vi "theOne_V3.vi"() -> ()   [LabVIEW 2021]
uses:
  <userlib>/er4commlib_labview/er4commlib_labview.lvlib
  <resource>/objmgr/nicontrollersysapi.rc
  <vilib>/nisyscfg/nisyscfg.lvlib
  <resource>/objmgr/nisysapi.rc
panel:
  in  "Tab Control 2":enum32{"const", "tri", "squa", "steps"}(tab)
  in  "Voltage Stimulus const":cluster{"stimulus":bool, "Vhold [mV]":dbl}={"stimulus"=FALSE, "Vhold [mV]"=-50.0} {"Vhold [mV]" format="%_5f"}
  in  "Voltage Stimulus tri":T1={"stimulus"=FALSE, "Vhold [mV]"=-50.0, "Vamp [mV]"=0.0, "Thold [ms]"=0.0} {"Thold [ms]" format="%_5f"; "Vamp [mV]" format="%_5f"; "Vhold [mV]" format="%_5f"}
  in  "Voltage Stimulus squa":T2={"stimulus"=FALSE, "Vhold [mV]"=-50.0, "Vpulse [mV]"=0.0, "Thold [ms]"=0.0, "Tpulse [ms]"=200.0} {"Tpulse [ms]" format="%_5f"; "Thold [ms]" format="%_5f"; "Vpulse [mV]" format="%_5f"; "Vhold [mV]" format="%_5f"}
  in  "Voltage Stimulus steps":T3={"stimulus"=FALSE, "Vhold [mV]"=-50.0, "Vpulse [mV]"=0.0, "Vstep [mV]"=10.0, "N"=10, "Thold [ms]"=0.0, "Tpulse [ms]"=200.0, "testVoff [mV]"=200.0, "testVoffCh"=127} {"testVoff [mV]" format="%_5f"; "Tpulse [ms]" format="%_5f"; "Thold [ms]" format="%_5f"; "Vstep [mV]" format="%_5f"; "Vpulse [mV]" format="%_5f"; "Vhold [mV]" format="%_5f"}
  out "Array 6":dbl[][](array[numeric])
  in  "save!":bool=TRUE
  out "actuall saving path":path
  out "refTxtSave":refnum<file>
  out "saving?":bool
  out "System Resources:Memory:Free Virtual":dbl=30432984.0
  in  "Target (localhost)":refnum<k21>="localhost"
  out "# elements to save":i32=45
  out "# elements to display":i32
  in  "save to":path=path "C:/temp/test.txt"
  out "DataCh1":dbl[](graph)
  out "DataCh2":dbl[](graph)
  out "DataCh3":dbl[](graph)
  out "DataCh4":dbl[](graph)
  out "VolAndTrig":dbl[][](graph)
  out "triggerImage":picture
  in  "path to triggerImage file jpg":path=path "C:/neoDiag/MrAnderson/Img/trigger.jpg"
  in  "Trigger":T4={"manual start"=FALSE, "duration [us]"=200.0, "period [ms]"=1.0, "delay [us]"=0.0, "reps"=1000, "active"=TRUE} {"delay [us]" format="%_5f"; "period [ms]" format="%_5f"; "duration [us]" format="%_5f"}
  in  "acquire data":bool
  in  "stop":bool
  out "pulseTrainImage":picture
  in  "path to pulseTrainImage file jpg":path=path "C:/neoDiag/MrAnderson/Img/volProtVarAmpl.jpg"
  in  "Tab Control":enum32{"AcqPara", "AdvPara"}(tab)
  in  "Acquisition Parameters":T5={"Camera "=FALSE, "Period [ms]"=200.0, "Duration [ms]"=0.2, "Delay [ms]"=0.0, "Pulses [#]"=10, "sampling rate [kHz]"="1,25", "current range [nA]"="2", "time display [s]"=0.5, "time recording [s]"=0.0} {"Delay [ms]" format="%_5f"; "Duration [ms]" format="%_5f"; "Period [ms]" format="%_5f"}
  in  "advancedSettings":T6={"Channels to read"=6, " dataPackets to read"=100, "displayRange"=625, "time acq loop [ms]"=25, "time rest loop [ms]"=25}
  out "Error Out Int":u32
  out "Error Out String":string="clean"
  out "E4 parameters":T7={"currentChannelsNum out"=1, "voltageChannelsNum out"=4, "gpChannelsNum out"=1, "sampling rate [kHz]"=1.25, "real sampling rate [kHz]"=1.220703125, "Ch_min"=-2.0, "Ch_max"=2.0, "Ch_step"=6.103701895199438e-05, "Ch_unit"=1e-09}
  in  "Display 1":cluster{"ChArray":bool[]}={"ChArray"=[FALSE, TRUE, TRUE, TRUE, FALSE, FALSE]}
  out "Error Read":errorcluster
  # "8MBit per element\ncan be improved setting min buffer of readData.vi"
  # "DataCh1"
  # "DataCh2"
  # "DataCh3"
  # "DataCh4"
  # "Voltage"
  # "Trigger"
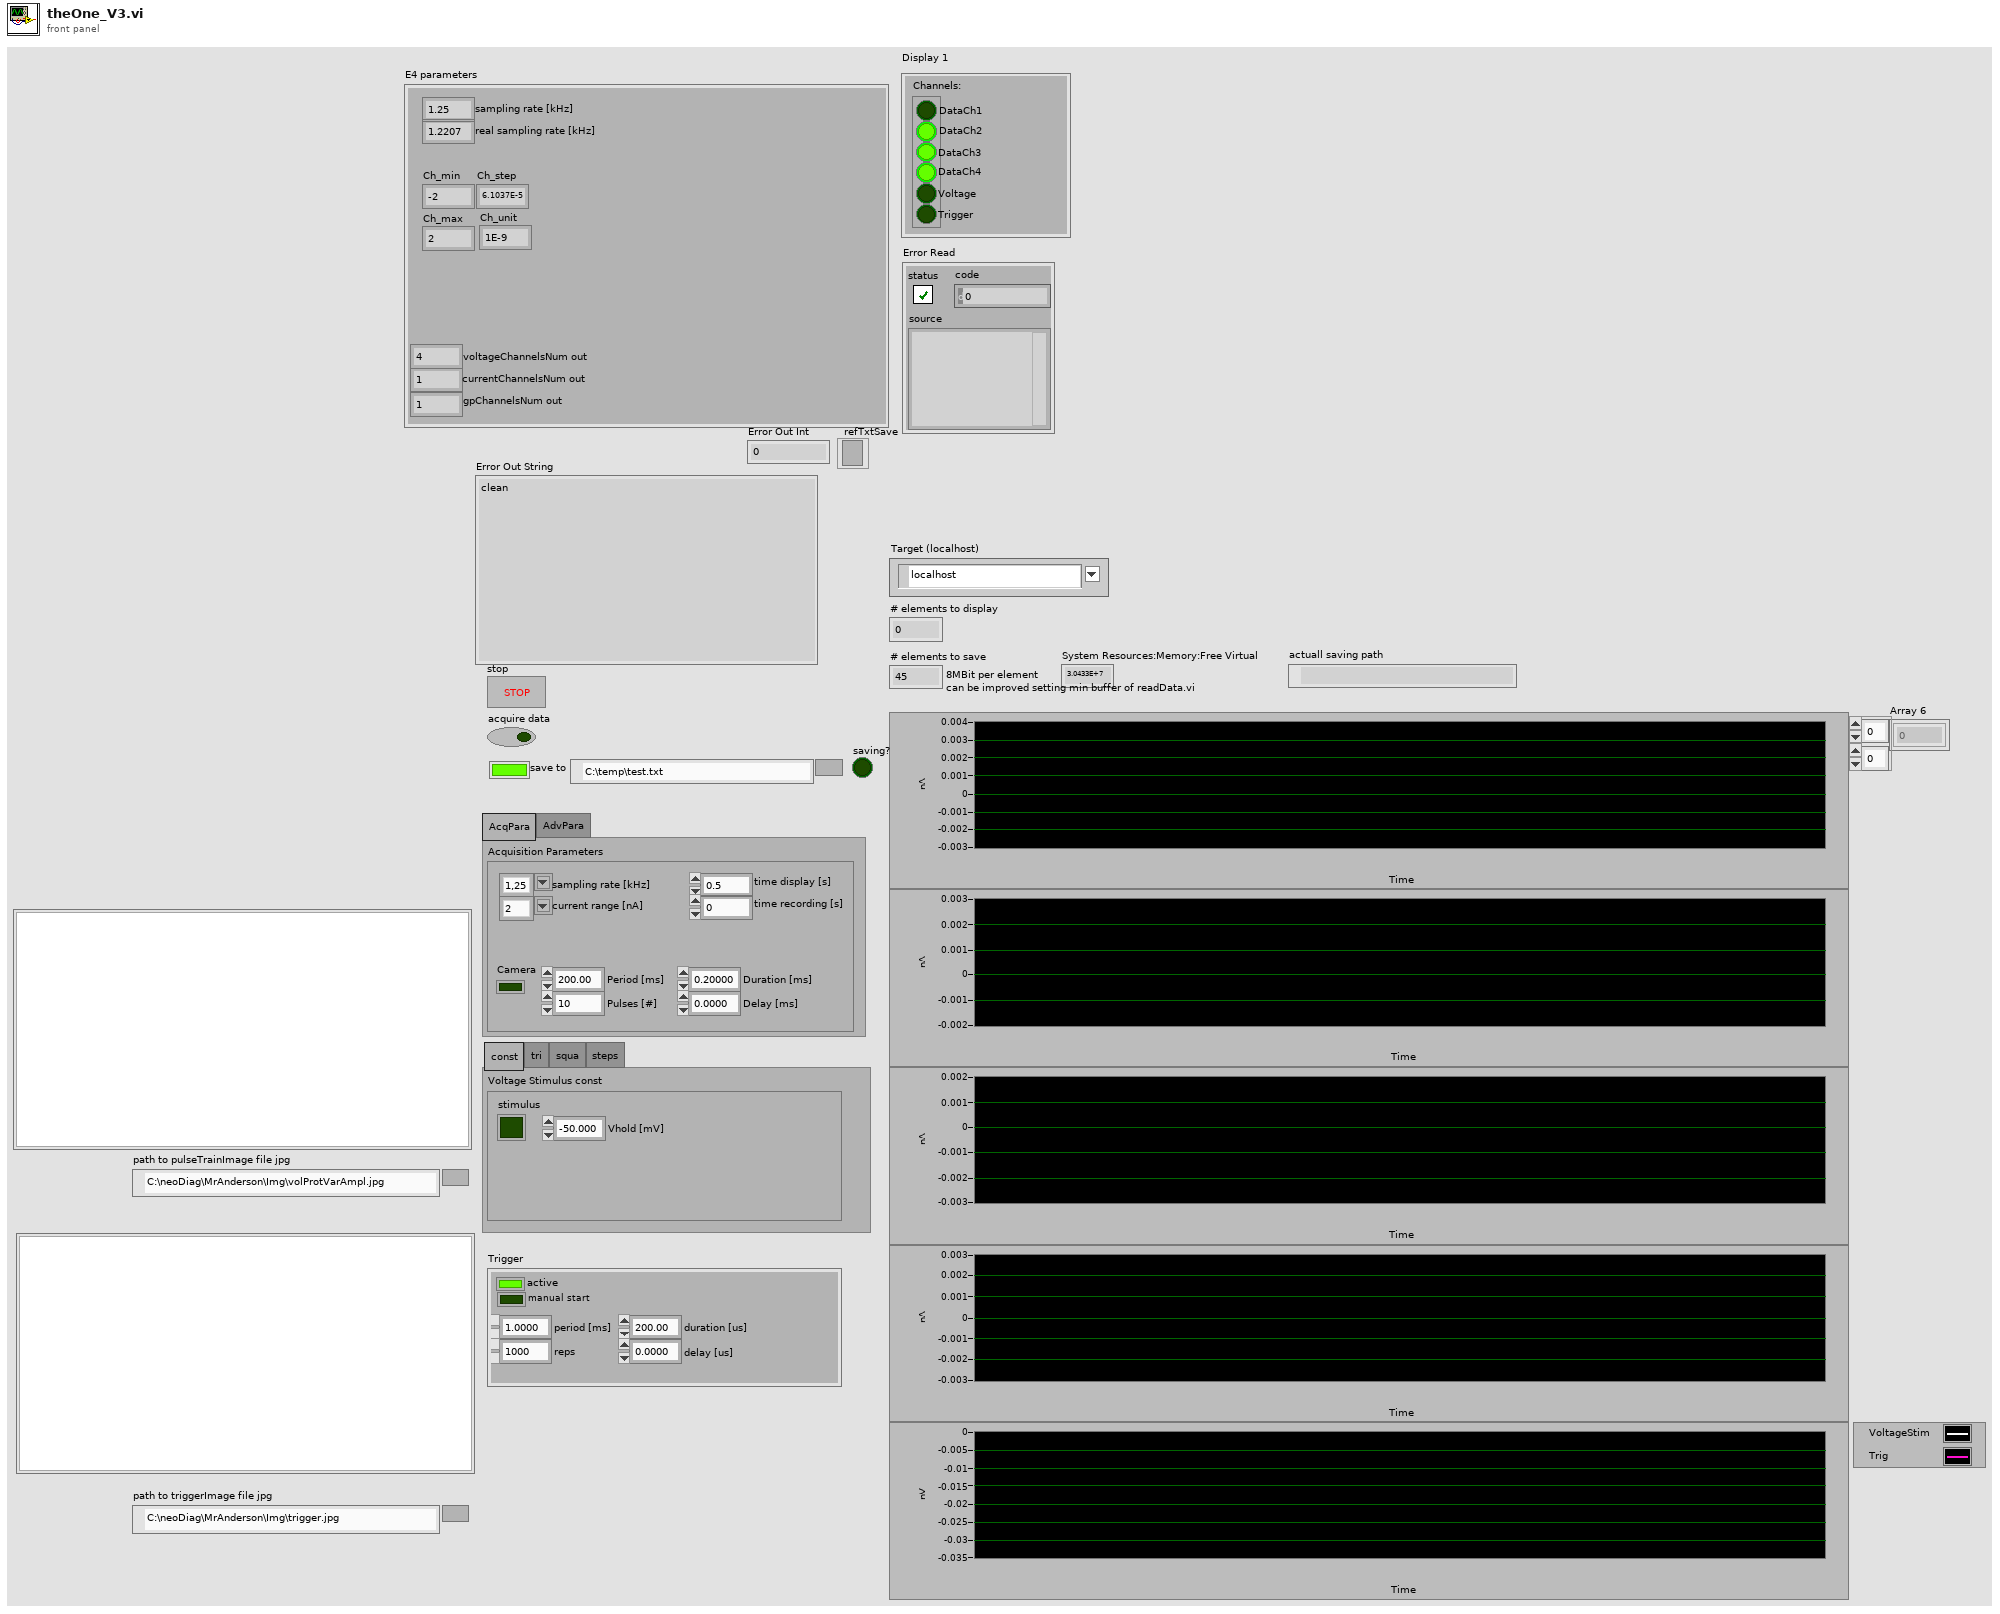
[diagram p1: front panel]
types:
  T1 = cluster{"stimulus":bool, "Vhold [mV]":dbl, "Vamp [mV]":dbl, "Thold [ms]":dbl}
  T2 = cluster{"stimulus":bool, "Vhold [mV]":dbl, "Vpulse [mV]":dbl, "Thold [ms]":dbl, "Tpulse [ms]":dbl}
  T3 = cluster{"stimulus":bool, "Vhold [mV]":dbl, "Vpulse [mV]":dbl, "Vstep [mV]":dbl, "N":u32, "Thold [ms]":dbl, "Tpulse [ms]":dbl, "testVoff [mV]":dbl, "testVoffCh":i8}
  T4 = cluster{"manual start":bool, "duration [us]":dbl, "period [ms]":dbl, "delay [us]":dbl, "reps":u32, "active":bool}
  T5 = cluster{"Camera ":bool, "Period [ms]":dbl, "Duration [ms]":dbl, "Delay [ms]":dbl, "Pulses [#]":u32, "sampling rate [kHz]":string, "current range [nA]":string, "time display [s]":dbl, "time recording [s]":dbl}
  T6 = cluster{"Channels to read":i32, " dataPackets to read":i32, "displayRange":i32, "time acq loop [ms]":u32, "time rest loop [ms]":u32}
  T7 = cluster{"currentChannelsNum out":u32, "voltageChannelsNum out":u32, "gpChannelsNum out":u32, "sampling rate [kHz]":dbl, "real sampling rate [kHz]":dbl, "Ch_min":dbl, "Ch_max":dbl, "Ch_step":dbl, "Ch_unit":dbl}
  T8 = cluster{"availableDataPackets":u32, "bufferOverflowFlag":bool, "lostDataFlag":bool, "saturationFlag":bool, "currentRangeIncreaseFlag":bool, "currentRangeDecreaseFlag":bool, "communicationErrorFlag":bool}
  T9 = enum16{"open", "replace", "create", "open or create", "replace or create", "replace or create with confirmation"}
  T10 = typedef "imagedata.ctl" = cluster{"image type":i32, "image depth":i32, "image":u8[], "mask":u8[], "colors":u32[], "Rectangle":cluster{"left":i16, "top":i16, "right":i16, "bottom":i16}}
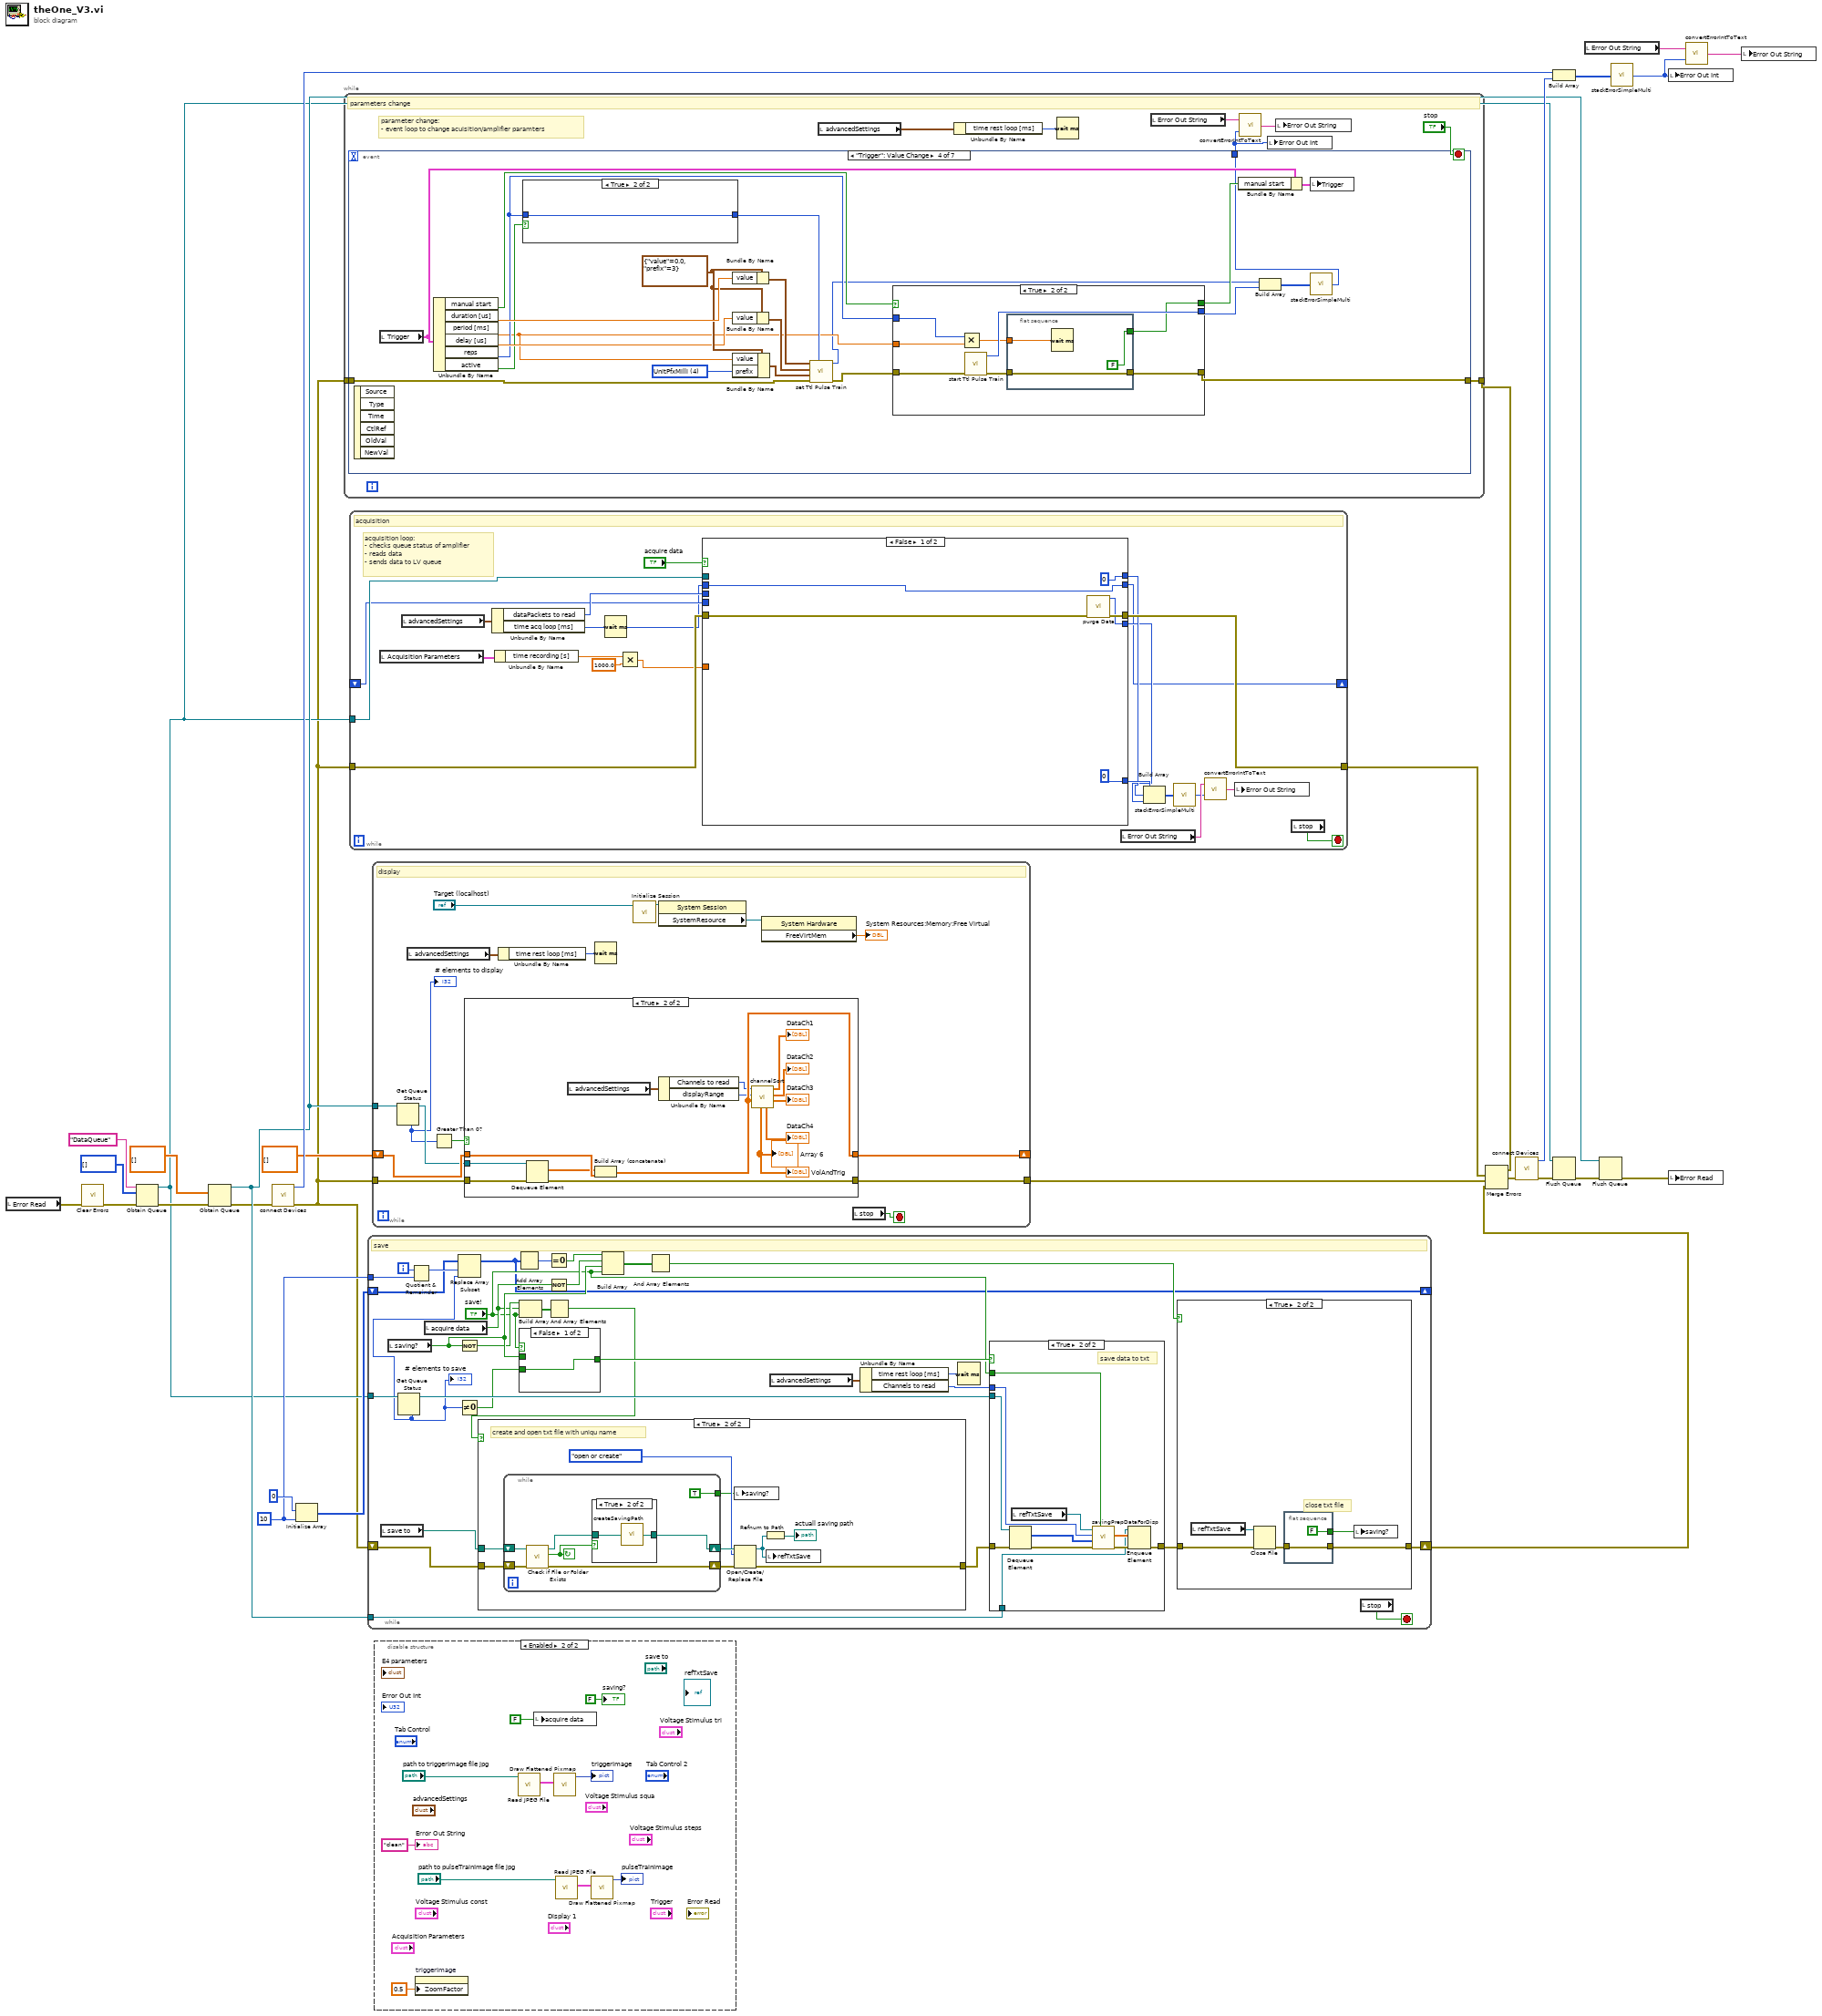
[diagram p0: block diagram]
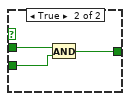
[diagram p2: hidden frame]
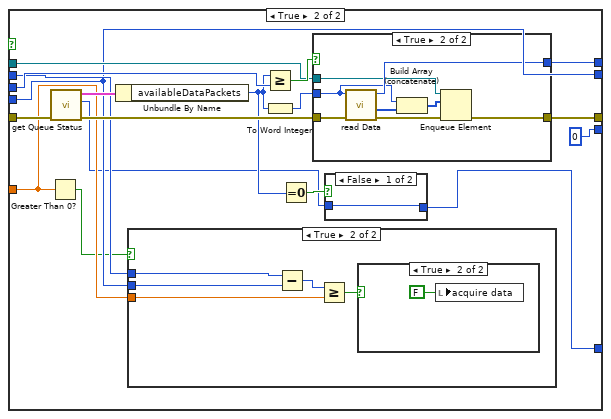
[diagram p8: hidden frame]
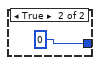
[diagram p9: hidden frame]
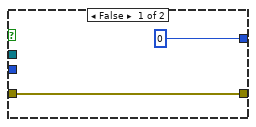
[diagram p12: hidden frame]
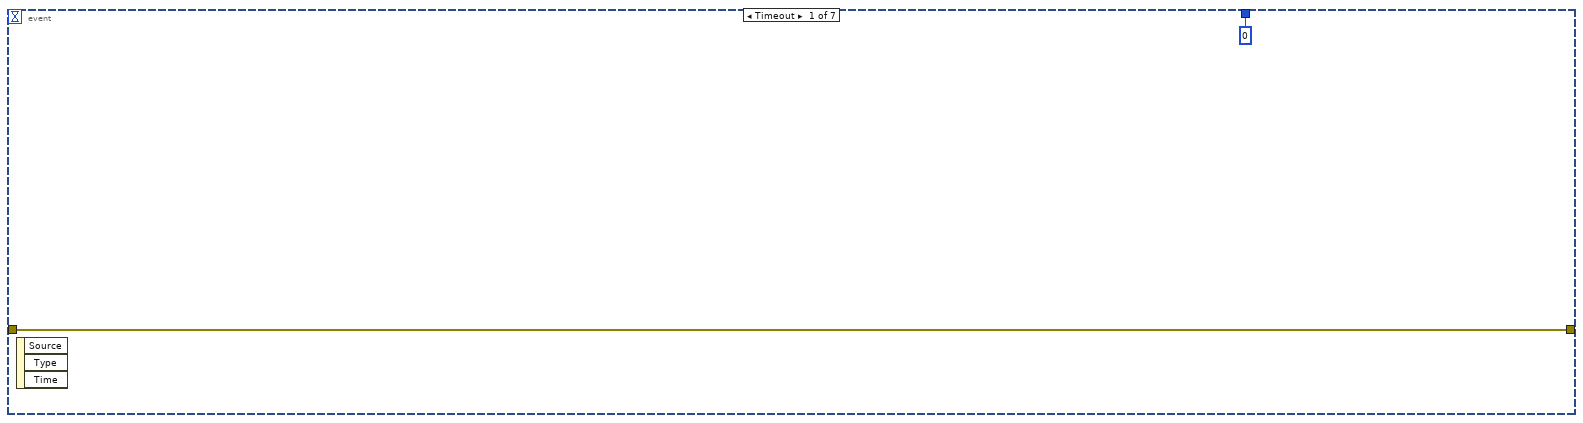
[diagram p13: hidden frame]
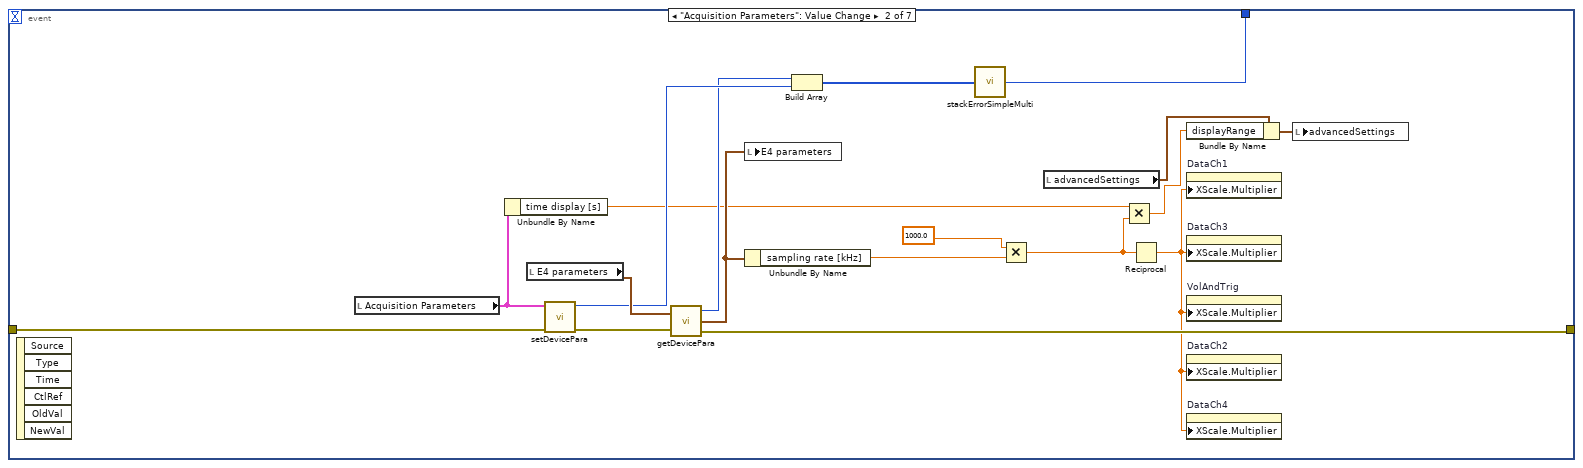
[diagram p14: hidden frame]
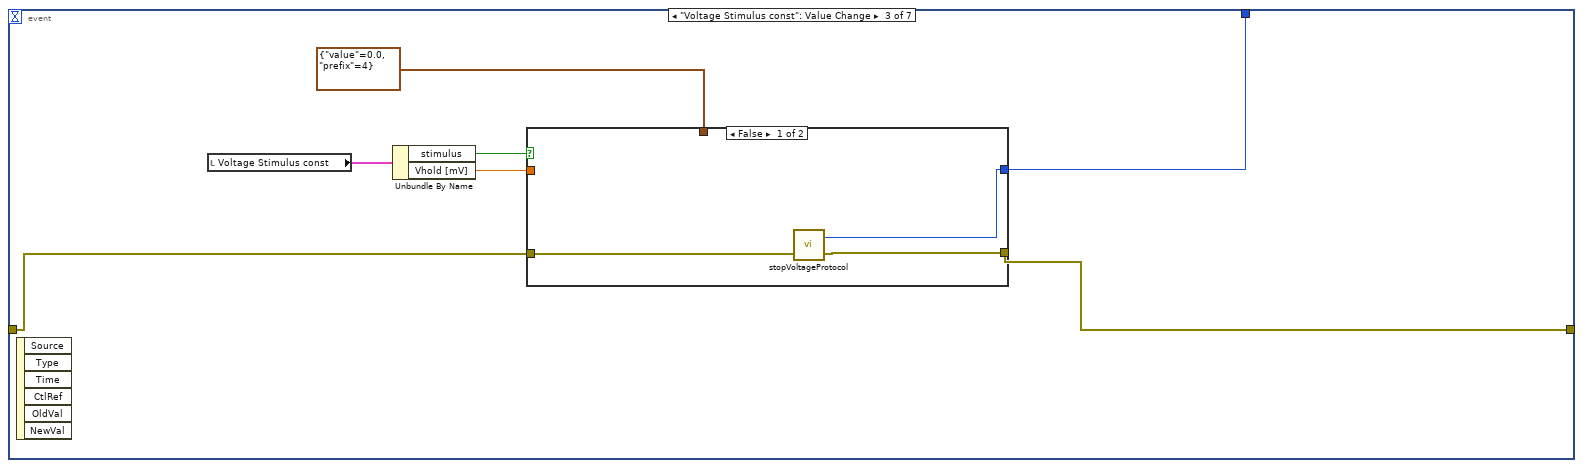
[diagram p15: hidden frame]
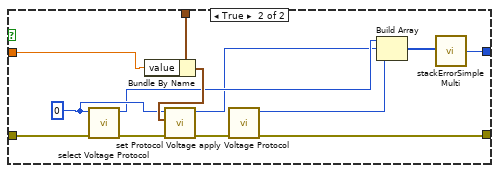
[diagram p16: hidden frame]
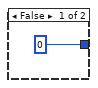
[diagram p17: hidden frame]
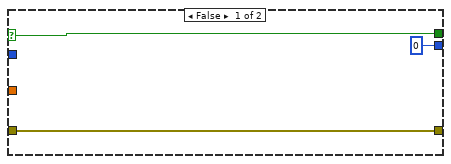
[diagram p18: hidden frame]
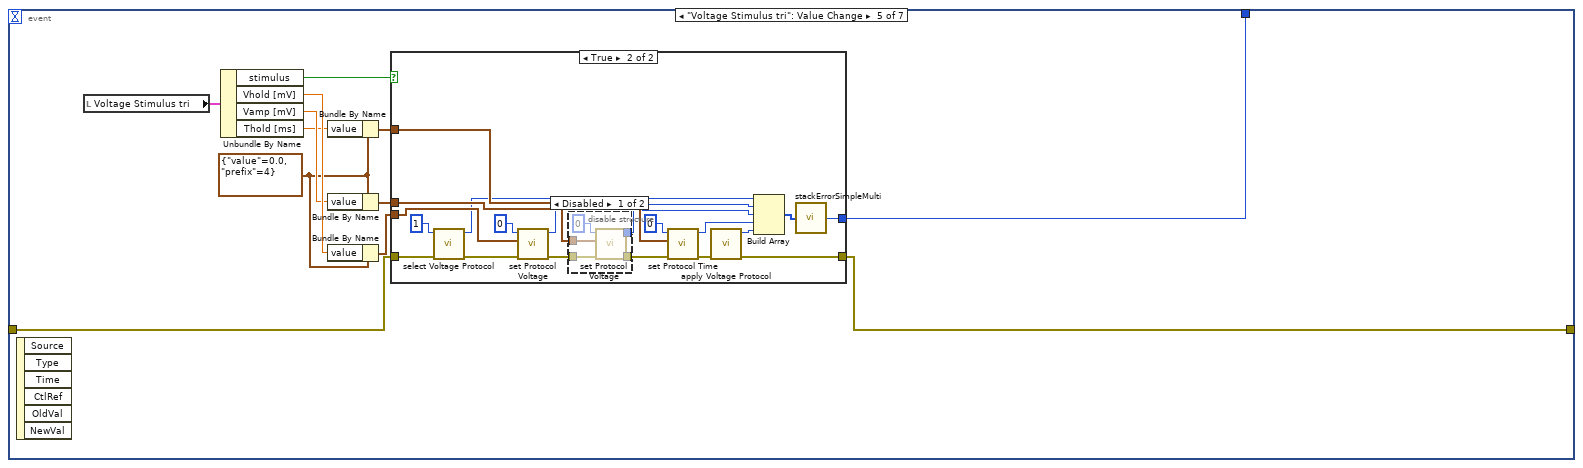
[diagram p19: hidden frame]
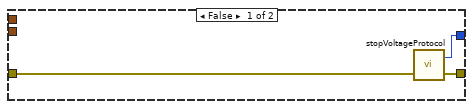
[diagram p20: hidden frame]
diagram:
  w3 = 10 ("dimension size")
  n1 = local read "Error Read"() -> (w28:errorcluster)
  n2 = call <vilib>:"Clear Errors.vi"("error in (no error)"=w28) -> ("error out"=w14:errorcluster)  [unwired: 5 in, 1 out]
  n3 = Obtain Queue(name (unnamed)="DataQueue", element data type=i16[] [] ("buffer out"), error in (no error)=w14) -> (queue out=w2:refnum<queue>, error out=w8:errorcluster)  [unwired: 2 in, 1 out]
  n4 = Obtain Queue(element data type=dbl[][] [] ("Array"), error in (no error)=w8) -> (queue out=w10:refnum<queue>, error out=w7:errorcluster)  [unwired: 3 in, 1 out]
  n5 = call <userlib>:"connect Devices.vi"("error in (no error)"=w7) -> ("error out"=w1:errorcluster, "function return"=w21:u32)  [unwired: 9 in]
  n6 = Initialize Array(0 ("dimension size"), w3) -> (w5:i32[])
  n7 = while {
    tunnel: w1 -> [w35]
    tunnel: [w34] -> w18
    stop <- "stop" stop-if-true
    # "parameter change:\n- event loop to change acuisition/amplifier paramters"
    # "parameters change"
    n8 = event shown="[3] \"Trigger\": Value Change" {
      selector: _ -> [_ _ _ _ _ _ _]
      dyn-events: _ -> [_ _ _ _ _ _ _]
      timeout: _ -> [_ _ _ _ _ _ _]
      tunnel: [w38 w51 w57 w100 w118 w160 w203] -> w34
      tunnel: w35 -> [w38 w50 w58 w92 w129 w170 w204]
      tunnel: [u32 0 ("function return") w39 w59 w80 w119 w161 w205] -> w29
      event Timeout {
        n9 = event-data() -> ()  [unwired: 1 in, 3 out]
      }
      event "Acquisition Parameters": Value Change {
        n10 = event-data() -> ()  [unwired: 1 in, 6 out]
        n11 = local read "Acquisition Parameters"() -> (w45:T5)
        n12 = Unbundle By Name(w45) -> ("time display [s]"=w44:dbl)
        n13 = local read "E4 parameters"() -> (w53:T7)
        n14 = call "setDevicePara.vi"("error in (no error)"=w50, "Acquisition Parameters"=w45) -> ("error out"=w55:errorcluster, "function return"=w49:u32)  [unwired: 8 in]
        n15 = call "getDevicePara.vi"("Seetings in"=w53, "error in (no error)"=w55) -> ("Error Out"=w48:u32, "Seetings out"=w54:T7, "error out"=w51:errorcluster)
        n16 = local write "E4 parameters"(w54) -> ()
        n17 = Unbundle By Name(w54) -> ("sampling rate [kHz]"=w56:dbl)
        n18 = Build Array(w48, w49) -> (w47:u32[])
        n19 = call "stackErrorSimpleMulti.vi"("Error List"=w47) -> ("Error Out"=w39:u32)
        n20 = Multiply(x=1000.0, y=w56) -> (x*y=w43:dbl)
        n21 = local read "advancedSettings"() -> (w40:T6)
        n22 = Multiply(x=w44, y=w43) -> (x*y=w41:dbl)
        n23 = Reciprocal(x=w43) -> (1/x=w46:dbl)
        n24 = Bundle By Name(cluster=w40, "displayRange"=w41) -> (w42:T6)
        n25 = property on="DataCh1" class="WFGraph (strict)"("XScale.Multiplier"=w46) -> ()  [unwired: 2 in, 2 out]
        n26 = property on="DataCh3" class="WFGraph (strict)"("XScale.Multiplier"=w46) -> ()  [unwired: 2 in, 2 out]
        n27 = property on="VolAndTrig" class="WFGraph (strict)"("XScale.Multiplier"=w46) -> ()  [unwired: 2 in, 2 out]
        n28 = property on="DataCh2" class="WFGraph (strict)"("XScale.Multiplier"=w46) -> ()  [unwired: 2 in, 2 out]
        n29 = property on="DataCh4" class="WFGraph (strict)"("XScale.Multiplier"=w46) -> ()  [unwired: 2 in, 2 out]
        n30 = local write "advancedSettings"(w42) -> ()
      }
      event "Voltage Stimulus const": Value Change {
        n31 = event-data() -> ()  [unwired: 1 in, 6 out]
        n32 = local read "Voltage Stimulus const"() -> (w63:cluster{"stimulus":bool, "Vhold [mV]":dbl})
        n33 = Unbundle By Name(w63) -> ("stimulus"=w62:bool, "Vhold [mV]"=w60:dbl)
        n34 = case shown="False" w62 {
          tunnel: cluster{"value":dbl, "prefix":u32} {"value"=0.0, "prefix"=4} ("pulseDuration") -> [_ w76]
          tunnel: w60 -> [_ w75]
          tunnel: w58 -> [w66 w74]
          tunnel: [w65 w73] -> w57
          tunnel: [w64 w67] -> w59
          frame False {
            n35 = call "stopVoltageProtocol.vi"("error in (no error)"=w66) -> ("error out"=w65:errorcluster, "Error Out"=w64:u32)  [unwired: 1 in]
          }
          frame True {
            w72 = u32 0 ("idx")
            n36 = call <userlib>:"select Voltage Protocol.vi"("error in (no error)"=w74, "idx"=w72) -> ("error out"=w77:errorcluster, "function return"=w71:u32)  [unwired: 8 in]
            n37 = Bundle By Name(cluster=w76, "value"=w75) -> (w78:cluster{"value":dbl, "prefix":u32})
            n38 = call <userlib>:"set Protocol Voltage.vi"("error in (no error)"=w77, "voltage"=w78, "idx"=w72) -> ("error out"=w79:errorcluster, "function return"=w70:u32)  [unwired: 7 in]
            n39 = call <userlib>:"apply Voltage Protocol.vi"("error in (no error)"=w79) -> ("error out"=w73:errorcluster, "function return"=w69:u32)  [unwired: 9 in]
            n40 = Build Array(w71, w70, w69) -> (w68:u32[])
            n41 = call "stackErrorSimpleMulti.vi"("Error List"=w68) -> ("Error Out"=w67:u32)
          }
        }
      }
      event "Trigger": Value Change {
        w95 = cluster{"value":dbl, "prefix":u32} {"value"=0.0, "prefix"=3} ("pulseDuration")
        w99 = u32 4 items=["UnitPfxFemto", "UnitPfxPico", "UnitPfxNano", "UnitPfxMicro", "UnitPfxMilli", "UnitPfxNone", "UnitPfxKilo", "UnitPfxMega", "UnitPfxGiga", "UnitPfxTera", "UnitPfxPeta", "UnitPfxNum"] ("prefix")
        n42 = event-data() -> ()  [unwired: 1 in, 6 out]
        n43 = local read "Trigger"() -> (w86:T4)
        n44 = Unbundle By Name(w86) -> ("manual start"=w101:bool, "duration [us]"=w97:dbl, "period [ms]"=w82:dbl, "delay [us]"=w94:dbl, "reps"=w83:u32, "active"=w90:bool)
        n45 = case shown="True" w90 {
          tunnel: w83 -> [_ w103]
          tunnel: [u32 0 ("reps") w103] -> w89
          frame False {
          }
          frame True {
          }
        }
        n46 = Bundle By Name(cluster=w95, "value"=w97) -> (w96:cluster{"value":dbl, "prefix":u32})
        n47 = Bundle By Name(cluster=w95, "value"=w94) -> (w93:cluster{"value":dbl, "prefix":u32})
        n48 = Bundle By Name(cluster=w95, "value"=w82, "prefix"=w99) -> (w98:cluster{"value":dbl, "prefix":u32})
        n49 = call <userlib>:"set Ttl Pulse Train.vi"("numberOfPulses"=w89, "error in (no error)"=w92, "period"=w98, "pulseDelay"=w93, "pulseDuration"=w96) -> ("error out"=w91:errorcluster, "function return"=w81:u32)  [unwired: 5 in]
        n50 = case shown="True" w101 {
          selector: w101 -> [w104 _]
          tunnel: w91 -> [w106 w114]
          tunnel: [w106 w110] -> w100
          tunnel: [u32 0 ("function return") w113] -> w87
          tunnel: [w104 w112] -> w85
          tunnel: w83 -> [_ w109]
          tunnel: w82 -> [_ w108]
          frame False {
          }
          frame True {
            n51 = Multiply(x=w109, y=w108) -> (x*y=w107:dbl)
            n52 = call <userlib>:"start Ttl Pulse Train.vi"("error in (no error)"=w114) -> ("error out"=w111:errorcluster, "function return"=w113:u32)  [unwired: 9 in]
            n53 = flat-sequence {
              tunnel: [FALSE] -> w112
              tunnel: w111 -> [w116]
              tunnel: [w116] -> w110
              tunnel: w107 -> [w115]
              frame #0 {
                n54 = Wait (ms)(milliseconds to wait=w115) -> ()  [unwired: 1 out]
              }
            }
          }
        }
        n55 = Bundle By Name(cluster=w86, "manual start"=w85) -> (w84:T4)
        n56 = Build Array(w81, w87) -> (w88:u32[])
        n57 = local write "Trigger"(w84) -> ()
        n58 = call "stackErrorSimpleMulti.vi"("Error List"=w88) -> ("Error Out"=w80:u32)
      }
      event "Voltage Stimulus tri": Value Change {
        w122 = cluster{"value":dbl, "prefix":u32} {"value"=0.0, "prefix"=4} ("frequency")
        n59 = event-data() -> ()  [unwired: 1 in, 6 out]
        n60 = local read "Voltage Stimulus tri"() -> (w128:T1)
        n61 = Unbundle By Name(w128) -> ("stimulus"=w127:bool, "Vhold [mV]"=w126:dbl, "Vamp [mV]"=w124:dbl, "Thold [ms]"=w121:dbl)
        n62 = Bundle By Name(cluster=w122, "value"=w121) -> (w120:cluster{"value":dbl, "prefix":u32})
        n63 = Bundle By Name(cluster=w122, "value"=w124) -> (w123:cluster{"value":dbl, "prefix":u32})
        n64 = Bundle By Name(cluster=w122, "value"=w126) -> (w125:cluster{"value":dbl, "prefix":u32})
        n65 = case shown="True" w127 {
          tunnel: w129 -> [w132 w151]
          tunnel: [w131 w149] -> w118
          tunnel: w125 -> [_ w147]
          tunnel: w123 -> [_ w143]
          tunnel: w120 -> [_ w142]
          tunnel: [w130 w134] -> w119
          frame False {
            n66 = call "stopVoltageProtocol.vi"("error in (no error)"=w132) -> ("error out"=w131:errorcluster, "Error Out"=w130:u32)  [unwired: 1 in]
          }
          frame True {
            n67 = call <userlib>:"select Voltage Protocol.vi"("error in (no error)"=w151, "idx"=u32 1) -> ("error out"=w150:errorcluster, "function return"=w137:u32)  [unwired: 8 in]
            n68 = call <userlib>:"set Protocol Voltage.vi"("error in (no error)"=w150, "voltage"=w147, "idx"=u32 0 ("N")) -> ("error out"=w146:errorcluster, "function return"=w139:u32)  [unwired: 7 in]
            n69 = disable-structure shown="Disabled" {
              disable-tunnel: w146 -> [w156 _]
              disable-tunnel: [w155 _] -> w145
              disable-tunnel: w143 -> [w154 _]
              disable-tunnel: [w152 _] -> w138
              frame Disabled {
                n70 = call <userlib>:"set Protocol Voltage.vi"("error in (no error)"=w156, "voltage"=w154, "idx"=u32 0 ("N")) -> ("error out"=w155:errorcluster, "function return"=w152:u32)  [unwired: 7 in]
              }
              frame Enabled {
              }
            }
            n71 = call <userlib>:"set Protocol Time.vi"("error in (no error)"=w145, "time"=w142, "idx"=u32 0 ("N")) -> ("error out"=w148:errorcluster, "function return"=w140:u32)  [unwired: 7 in]
            n72 = call <userlib>:"apply Voltage Protocol.vi"("error in (no error)"=w148) -> ("error out"=w149:errorcluster, "function return"=w136:u32)  [unwired: 9 in]
            n73 = Build Array(w137, w139, w138, w140, w136) -> (w135:u32[])
            n74 = call "stackErrorSimpleMulti.vi"("Error List"=w135) -> ("Error Out"=w134:u32)
          }
        }
      }
      event "Voltage Stimulus squa": Value Change {
        w157 = cluster{"value":dbl, "prefix":u32} {"value"=0.0, "prefix"=4} ("frequency")
        n75 = event-data() -> ()  [unwired: 1 in, 6 out]
        n76 = local read "Voltage Stimulus squa"() -> (w169:T2)
        n77 = Unbundle By Name(w169) -> ("stimulus"=w168:bool, "Vhold [mV]"=w167:dbl, "Vpulse [mV]"=w165:dbl, "Thold [ms]"=w163:dbl, "Tpulse [ms]"=w159:dbl)
        n78 = Bundle By Name(cluster=w157, "value"=w159) -> (w158:cluster{"value":dbl, "prefix":u32})
        n79 = Bundle By Name(cluster=w157, "value"=w163) -> (w162:cluster{"value":dbl, "prefix":u32})
        n80 = Bundle By Name(cluster=w157, "value"=w165) -> (w164:cluster{"value":dbl, "prefix":u32})
        n81 = Bundle By Name(cluster=w157, "value"=w167) -> (w166:cluster{"value":dbl, "prefix":u32})
        n82 = case shown="True" w168 {
          tunnel: w170 -> [w173 w197]
          tunnel: [w172 w195] -> w160
          tunnel: w166 -> [_ w194]
          tunnel: w164 -> [_ w190]
          tunnel: w162 -> [_ w189]
          tunnel: [w171 w182] -> w161
          tunnel: w158 -> [_ w179]
          frame False {
            n83 = call "stopVoltageProtocol.vi"("error in (no error)"=w173) -> ("error out"=w172:errorcluster, "Error Out"=w171:u32)  [unwired: 1 in]
          }
          frame True {
            n84 = call <userlib>:"select Voltage Protocol.vi"("error in (no error)"=w197, "idx"=u32 2) -> ("error out"=w196:errorcluster, "function return"=w184:u32)  [unwired: 8 in]
            n85 = call <userlib>:"set Protocol Voltage.vi"("error in (no error)"=w196, "voltage"=w194, "idx"=u32 0 ("N")) -> ("error out"=w193:errorcluster, "function return"=w186:u32)  [unwired: 7 in]
            n86 = call <userlib>:"set Protocol Voltage.vi"("error in (no error)"=w193, "voltage"=w190, "idx"=u32 1 ("N")) -> ("error out"=w192:errorcluster, "function return"=w185:u32)  [unwired: 7 in]
            n87 = call <userlib>:"set Protocol Time.vi"("error in (no error)"=w192, "time"=w189, "idx"=u32 0 ("N")) -> ("error out"=w178:errorcluster, "function return"=w187:u32)  [unwired: 7 in]
            n88 = call <userlib>:"set Protocol Time.vi"("error in (no error)"=w178, "time"=w179, "idx"=u32 1) -> ("error out"=w176:errorcluster, "function return"=w175:u32)  [unwired: 7 in]
            n89 = call <userlib>:"apply Voltage Protocol.vi"("error in (no error)"=w176) -> ("error out"=w195:errorcluster, "function return"=w174:u32)  [unwired: 9 in]
            n90 = Build Array(w184, w186, w185, w187, w175, w174) -> (w183:u32[])
            n91 = call "stackErrorSimpleMulti.vi"("Error List"=w183) -> ("Error Out"=w182:u32)
          }
        }
      }
      event "Voltage Stimulus steps": Value Change {
        n92 = event-data() -> ()  [unwired: 1 in, 6 out]
        n93 = disable-structure shown="Disabled" {
          disable-tunnel: w204 -> [w219 _]
          disable-tunnel: [w210 _] -> w205
          disable-tunnel: [w209 _] -> _
          frame Disabled {
            w206 = cluster{"value":dbl, "prefix":u32} {"value"=0.0, "prefix"=4} ("frequency")
            n94 = local read "Voltage Stimulus steps"() -> (w218:T3)
            n95 = Unbundle By Name(w218) -> ("stimulus"=w217:bool, "Vhold [mV]"=w216:dbl, "Vpulse [mV]"=w214:dbl, "Thold [ms]"=w212:dbl, "Tpulse [ms]"=w208:dbl)
            n96 = Bundle By Name(cluster=w206, "value"=w208) -> (w207:cluster{"value":dbl, "prefix":u32})
            n97 = Bundle By Name(cluster=w206, "value"=w212) -> (w211:cluster{"value":dbl, "prefix":u32})
            n98 = Bundle By Name(cluster=w206, "value"=w214) -> (w213:cluster{"value":dbl, "prefix":u32})
            n99 = Bundle By Name(cluster=w206, "value"=w216) -> (w215:cluster{"value":dbl, "prefix":u32})
            n100 = case shown="True" w217 {
              tunnel: w219 -> [w222 w246]
              tunnel: [w221 w244] -> w209
              tunnel: w215 -> [_ w243]
              tunnel: w213 -> [_ w239]
              tunnel: w211 -> [_ w238]
              tunnel: [w220 w231] -> w210
              tunnel: w207 -> [_ w228]
              frame False {
                n101 = call "stopVoltageProtocol.vi"("error in (no error)"=w222) -> ("error out"=w221:errorcluster, "Error Out"=w220:u32)  [unwired: 1 in]
              }
              frame True {
                n102 = call <userlib>:"select Voltage Protocol.vi"("error in (no error)"=w246, "idx"=u32 2) -> ("error out"=w245:errorcluster, "function return"=w233:u32)  [unwired: 8 in]
                n103 = call <userlib>:"set Protocol Voltage.vi"("error in (no error)"=w245, "voltage"=w243, "idx"=u32 0 ("N")) -> ("error out"=w242:errorcluster, "function return"=w235:u32)  [unwired: 7 in]
                n104 = call <userlib>:"set Protocol Voltage.vi"("error in (no error)"=w242, "voltage"=w239, "idx"=u32 1 ("N")) -> ("error out"=w241:errorcluster, "function return"=w234:u32)  [unwired: 7 in]
                n105 = call <userlib>:"set Protocol Time.vi"("error in (no error)"=w241, "time"=w238, "idx"=u32 0 ("N")) -> ("error out"=w227:errorcluster, "function return"=w236:u32)  [unwired: 7 in]
                n106 = call <userlib>:"set Protocol Time.vi"("error in (no error)"=w227, "time"=w228, "idx"=u32 1) -> ("error out"=w225:errorcluster, "function return"=w224:u32)  [unwired: 7 in]
                n107 = call <userlib>:"apply Voltage Protocol.vi"("error in (no error)"=w225) -> ("error out"=w244:errorcluster, "function return"=w223:u32)  [unwired: 9 in]
                n108 = Build Array(w233, w235, w234, w236, w224, w223) -> (w232:u32[])
                n109 = call "stackErrorSimpleMulti.vi"("Error List"=w232) -> ("Error Out"=w231:u32)
              }
            }
          }
          frame Enabled {
          }
        }
        n110 = local read "Voltage Stimulus steps"() -> (w202:T3)
        n111 = Unbundle By Name(w202) -> ("testVoffCh"=w201:i8, "testVoff [mV]"=w200:dbl)
        n112 = Bundle By Name(cluster=cluster{"value":dbl, "prefix":u32} {"value"=0.0, "prefix"=4} ("frequency"), "value"=w200) -> (w198:cluster{"value":dbl, "prefix":u32})
        n113 = call <userlib>:"set Voltage Offset.vi"("error in (no error)"=w204, "voltage"=w198, "channelIdx"=w201) -> ("error out"=w203:errorcluster)  [unwired: 7 in, 1 out]
      }
    }
    n114 = local read "advancedSettings"() -> (w32:T6)
    n115 = Unbundle By Name(w32) -> ("time rest loop [ms]"=w33:u32)
    n116 = Wait (ms)(milliseconds to wait=w33) -> ()  [unwired: 1 out]
    n117 = local read "Error Out String"() -> (w31:string)
    n118 = call "convertErrorIntToText.vi"("Error Int In (function return)"=w29, "Error String In"=w31) -> ("Error String Out"=w30:string)
    n119 = local write "Error Out Int"(w29) -> ()
    n120 = local write "Error Out String"(w30) -> ()
  }
  n121 = while {
    tunnel: w1 -> [w267]
    tunnel: [w266] -> w17
    tunnel: w2 -> [w265]
    shift-right: [w250] -> _
    shift-left: _ -> [w249]
    stop <- w268 stop-if-true
    # "acquisition loop:\n- checks queue status of amplifier\n- reads data\n- sends data to LV queue"
    # "acquisition"
    n122 = local read "Acquisition Parameters"() -> (w254:T5)
    n123 = local read "advancedSettings"() -> (w257:T6)
    n124 = Unbundle By Name(w257) -> ("dataPackets to read"=w256:i32, "time acq loop [ms]"=w255:u32)
    n125 = Unbundle By Name(w254) -> ("time recording [s]"=w253:dbl)
    n126 = Wait (ms)(milliseconds to wait=w255) -> (millisecond timer value=w248:u32)
    n127 = Multiply(x=w253, y=1000.0) -> (x*y=w252:dbl)
    n128 = case shown="False" "acquire data" {
      tunnel: w267 -> [w269 w290]
      tunnel: [w274 w289] -> w266
      tunnel: w265 -> [_ w284]
      tunnel: [u32 0 ("function return") w276] -> w260
      tunnel: [u32 0 ("function return") w287] -> w259
      tunnel: [w273 u32 0 ("function return")] -> w258
      tunnel: w256 -> [_ w285]
      tunnel: w252 -> [_ w280]
      tunnel: w248 -> [w270 w282]
      tunnel: [w270 w281] -> w250
      tunnel: w249 -> [_ w281]
      frame False {
        n129 = call <userlib>:"purge Data.vi"("error in (no error)"=w269) -> ("error out"=w274:errorcluster, "function return"=w273:u32)  [unwired: 9 in]
      }
      frame True {
        n130 = Greater Than 0?(x=w280) -> (x > 0?=w275:bool)
        n131 = call <userlib>:"get Queue Status.vi"("error in (no error)"=w290) -> ("error out"=w291:errorcluster, "function return"=w277:u32, "status out"=w292:T8)  [unwired: 8 in]
        n132 = Unbundle By Name(w292) -> ("availableDataPackets"=w278:u32)
        n133 = case shown="True" w275 {
          tunnel: w280 -> [_ w299]
          tunnel: w282 -> [_ w296]
          tunnel: w281 -> [_ w295]
          frame False {
          }
          frame True {
            n134 = Subtract(x=w296, y=w295) -> (x-y=w297:u32)
            n135 = Greater Or Equal?(x=w297, y=w299) -> (x >= y?=w298:bool)
            n136 = case shown="True" w298 {
              frame False {
              }
              frame True {
                n137 = local write "acquire data"(FALSE ("acquire data")) -> ()
              }
            }
          }
        }
        n138 = Greater Or Equal?(x=w278, y=w285) -> (x >= y?=w288:bool)
        n139 = To Word Integer(number=w278) -> (16bit integer=w283:i16)
        n140 = Equal To 0?(x=w278) -> (x = 0?=w279:bool)
        n141 = case shown="True" w288 {
          tunnel: w291 -> [w302 w310]
          tunnel: w283 -> [_ w306]
          tunnel: [w302 w304] -> w289
          tunnel: [u32 0 ("function return") w309] -> w287
          tunnel: w284 -> [_ w308]
          frame False {
          }
          frame True {
            n142 = call <userlib>:"read Data.vi"("error in (no error)"=w310, "dataToRead"=w306) -> ("error out"=w305:errorcluster, "buffer out"=w307:i16[], "function return"=w309:u32)  [unwired: 6 in, 1 out]
            n143 = Build Array (concatenate)(w306, w307) -> (w303:i16[])
            n144 = Enqueue Element(queue=w308, element=w303, error in (no error)=w305) -> (error out=w304:errorcluster)  [unwired: 1 in, 2 out]
          }
        }
        n145 = case shown="False" w279 {
          tunnel: w277 -> [w293 _]
          tunnel: [w293 u32 0 ("function return")] -> w276
          frame False {
          }
          frame True {
          }
        }
      }
    }
    n146 = local read "Error Out String"() -> (w263:string)
    n147 = Build Array(w260, w259, w258) -> (w262:u32[])
    n148 = call "stackErrorSimpleMulti.vi"("Error List"=w262) -> ("Error Out"=w261:u32)
    n149 = call "convertErrorIntToText.vi"("Error Int In (function return)"=w261, "Error String In"=w263) -> ("Error String Out"=w264:string)
    n150 = local write "Error Out String"(w264) -> ()
    n151 = local read "stop"() -> (w268:bool)
  }
  n152 = while {
    tunnel: w2 -> [w336]
    tunnel: w10 -> [w312]
    tunnel: w3 -> [w340]
    shift-right: [w341] -> w6
    shift-left: w1 -> [w329]
    shift-right: [w311] -> _
    shift-left: w5 -> [w316]
    i -> [w337]
    stop <- w339 stop-if-true
    # "save"
    n153 = local read "save to"() -> (w328:path)
    n154 = local read "saving?"() -> (w322:bool)
    n155 = Get Queue Status(queue=w336) -> (queue out=w335:refnum<queue>, # elements in queue=w315:i32)  [unwired: 2 in, 6 out]
    "# elements to save" <- w315
    n156 = Quotient & Remainder(x=w337, y=w340) -> (x-y*floor(x/y)=w332:i32)  [unwired: 1 out]
    n157 = local read "acquire data"() -> (w318:bool)
    n158 = Replace Array Subset(array=w316, new element=w315, index=w332) -> (w311:i32[])
    n159 = Not(x=w322) -> (.not. x?=w320:bool)
    n160 = Not Equal To 0?(x=w315) -> (x != 0?=w330:bool)
    n161 = Add Array Elements(numeric array=w311) -> (sum=w333:i32)
    n162 = Build Array(w320, w318, "save!") -> (w319:bool[])
    n163 = case shown="False" "save!" {
      tunnel: [w342 w345] -> w331
      tunnel: w330 -> [w342 w344]
      tunnel: w322 -> [_ w343]
      frame False {
      }
      frame True {
        n164 = And(x=w343, y=w344) -> (x .and. y?=w345:bool)
      }
    }
    n165 = Equal To 0?(x=w333) -> (x = 0?=w326:bool)
    n166 = Not(x=w318) -> (.not. x?=w325:bool)
    n167 = And Array Elements(Boolean array=w319) -> (logical AND=w313:bool)
    n168 = case shown="True" w313 {
      tunnel: w328 -> [_ w373]
      tunnel: w329 -> [w366 w375]
      tunnel: [w366 w374] -> w314
      frame False {
      }
      frame True {
        # "create and open txt file with uniqu name"
        n169 = while {
          shift-right: [w380] -> w372
          shift-left: w375 -> [w382]
          shift-right: [w378] -> w371
          shift-left: w373 -> [w381]
          tunnel: [TRUE ("saving? 2")] -> w369
          stop <- w377 continue-if-true
          n170 = call <vilib>:"Check if File or Folder Exists.vi"("error in (no error)"=w382, "path"=w381) -> ("error out"=w380:errorcluster, "file or folder exists?"=w377:bool, "dup path"=w379:path)  [unwired: 7 in]
          n171 = case shown="True" w377 {
            tunnel: w379 -> [w383 w385]
            tunnel: [w383 w384] -> w378
            frame False {
            }
            frame True {
              n172 = call "createSavingPath.vi"("pathIn"=w385) -> ("pathOut"=w384:path)
            }
          }
        }
        n173 = local write "saving?"(w369) -> ()
        n174 = Open/Create/Replace File(file path (use dialog)=w371, error in=w372, operation (0:open)=T9."open or create") -> (refnum out=w368:refnum<file>, error out=w374:errorcluster)  [unwired: 3 in, 1 out]
        n175 = Refnum to Path(1:w368) -> (0:→"actuall saving path":path)
        n176 = local write "refTxtSave"(w368) -> ()
      }
    }
    n177 = Build Array(w326, w325, w322, "save!") -> (w324:bool[])
    n178 = And Array Elements(Boolean array=w324) -> (logical AND=w323:bool)
    n179 = local read "advancedSettings"() -> (w338:T6)
    n180 = Unbundle By Name(w338) -> ("time rest loop [ms]"=w334:u32, "Channels to read"=w321:i32)
    n181 = Wait (ms)(milliseconds to wait=w334) -> ()  [unwired: 1 out]
    n182 = case shown="True" w331 {
      tunnel: [w354 w359] -> w327
      tunnel: w335 -> [_ w365]
      tunnel: w314 -> [w354 w361]
      tunnel: w321 -> [_ w357]
      tunnel: "save!" -> [_ w356]
      tunnel: w312 -> [_ w355]
      frame False {
      }
      frame True {
        # "save data to txt"
        n183 = Dequeue Element(queue=w365, error in (no error)=w361) -> (element=w364:i16[], error out=w362:errorcluster)  [unwired: 1 in, 2 out]
        n184 = local read "refTxtSave"() -> (w358:refnum<file>)
        n185 = call "savingPrepDataForDisp.vi"("save"=w356, "error in (no error)"=w362, "buffer in"=w364, "Channels to read"=w357, "Byte Stream File in"=w358) -> ("error out"=w360:errorcluster, "Array"=w363:dbl[][])  [unwired: 4 in, 1 out]
        n186 = Enqueue Element(queue=w355, element=w363, error in (no error)=w360) -> (error out=w359:errorcluster)  [unwired: 1 in, 2 out]
      }
    }
    n187 = case shown="True" w323 {
      tunnel: [w346 w348] -> w341
      tunnel: w327 -> [w346 w351]
      frame False {
      }
      frame True {
        # "close txt file"
        n188 = local read "refTxtSave"() -> (w350:refnum<file>)
        n189 = Close File(refnum=w350, error in=w351) -> (error out=w349:errorcluster)  [unwired: 1 out]
        n190 = flat-sequence {
          tunnel: w349 -> [w353]
          tunnel: [w353] -> w348
          tunnel: [FALSE ("readyTosav")] -> w347
          frame #0 {
          }
        }
        n191 = local write "saving?"(w347) -> ()
      }
    }
    n192 = local read "stop"() -> (w339:bool)
  }
  n193 = while {
    tunnel: w1 -> [w400]
    tunnel: [w399] -> w13
    shift-right: [w398] -> _
    shift-left: dbl[][] [] ("Array") -> [w397]
    tunnel: w10 -> [w391]
    stop <- w396 stop-if-true
    # "display"
    n194 = Get Queue Status(queue=w391) -> (queue out=w395:refnum<queue>, # elements in queue=w394:i32)  [unwired: 2 in, 6 out]
    "# elements to display" <- w394
    n195 = local read "advancedSettings"() -> (w393:T6)
    n196 = Greater Than 0?(x=w394) -> (x > 0?=w390:bool)
    n197 = case shown="True" w390 {
      tunnel: w400 -> [w401 w404]
      tunnel: [w401 w403] -> w399
      tunnel: [w402 w415] -> w398
      tunnel: w397 -> [w402 w406]
      tunnel: w395 -> [_ w412]
      frame False {
      }
      frame True {
        n198 = Dequeue Element(queue=w412, error in (no error)=w404) -> (element=w405:dbl[][], error out=w403:errorcluster)  [unwired: 1 in, 2 out]
        n199 = local read "advancedSettings"() -> (w416:T6)
        n200 = Build Array (concatenate)(w405, w406) -> (w415:dbl[][])
        n201 = Unbundle By Name(w416) -> ("Channels to read"=w413:i32, "displayRange"=w414:i32)
        n202 = call "channelSort.vi"("Array 7"=w415, "displayRange"=w414, "Channels to read"=w413) -> ("Array 4"=→"DataCh3":dbl[], "Array 3"=→"DataCh2":dbl[], "Array 2"=→"DataCh1":dbl[], "Array 5"=→"DataCh4":dbl[], "Array 6"=→"VolAndTrig" →"Array 6":dbl[][])  [unwired: 3 in, 1 out]
      }
    }
    n203 = Unbundle By Name(w393) -> ("time rest loop [ms]"=w392:u32)
    n204 = Wait (ms)(milliseconds to wait=w392) -> ()  [unwired: 1 out]
    n205 = call <vilib>:"Initialize Session.vi"("Target (localhost)"="Target (localhost)") -> ("Session out"=w388:refnum<k21>)  [unwired: 9 in, 1 out]
    n206 = property class="System Session"(reference=w388) -> ("SystemResource"=w387:refnum<k20>)  [unwired: 1 in, 2 out]
    n207 = property class="System Hardware"(reference=w387) -> ("FreeVirtMem"=→"System Resources:Memory:Free Virtual":dbl)  [unwired: 1 in, 2 out]
    n208 = local read "stop"() -> (w396:bool)
  }
  n209 = disable-structure shown="Enabled" {
    frame Disabled {
    }
    frame Enabled {
      n210 = property on="triggerImage" class="Pict"("ZoomFactor"=sgl 0.5 ("Zoom Factor")) -> ()  [unwired: 2 in, 2 out]
      n211 = call <vilib>:"Read JPEG File.vi"("path to JPEG file"="path to triggerImage file jpg") -> ("image data"=w422:T10)  [unwired: 8 in, 2 out]
      n212 = local write "acquire data"(FALSE ("acquire data")) -> ()
      n213 = call <vilib>:"Draw Flattened Pixmap.vi"("image data"=w422) -> ("new picture"=→"triggerImage":picture)  [unwired: 8 in]
      n214 = call <vilib>:"Read JPEG File.vi"("path to JPEG file"="path to pulseTrainImage file jpg") -> ("image data"=w425:T10)  [unwired: 8 in, 2 out]
      n215 = call <vilib>:"Draw Flattened Pixmap.vi"("image data"=w425) -> ("new picture"=→"pulseTrainImage":picture)  [unwired: 8 in]
      "Error Out String" <- "clean" ("Error String Out")
      "saving?" <- FALSE ("saving? 2")
    }
  }
  n216 = Merge Errors(w18, w17, w13, w6) -> (w27:errorcluster)
  n217 = call <userlib>:"connect Devices.vi"("error in (no error)"=w27) -> ("error out"=w12:errorcluster, "function return"=w23:u32)  [unwired: 9 in]
  n218 = Build Array(w21, w23) -> (w25:u32[])
  n219 = Flush Queue(queue=w2, error in (no error)=w12) -> (error out=w11:errorcluster)  [unwired: 2 out]
  n220 = local read "Error Out String"() -> (w22:string)
  n221 = Flush Queue(queue=w10, error in (no error)=w11) -> (error out=w9:errorcluster)  [unwired: 2 out]
  n222 = call "stackErrorSimpleMulti.vi"("Error List"=w25) -> ("Error Out"=w26:u32)
  n223 = local write "Error Out Int"(w26) -> ()
  n224 = local write "Error Read"(w9) -> ()
  n225 = call "convertErrorIntToText.vi"("Error Int In (function return)"=w26, "Error String In"=w22) -> ("Error String Out"=w24:string)
  n226 = local write "Error Out String"(w24) -> ()
